vi "Handle Command.vi"(8 "error in":errorcluster, 10 "Change TEC SPs in":refnum<class "Change TEC SPs.lvclass">, 11 "Object In":refnum<class>) -> (0 "error out":errorcluster, 1 "Command Successful?":bool, 2 "Change TEC SPs out":refnum<class "Change TEC SPs.lvclass">, 3 "Object Out":refnum<class>)   [LabVIEW 2014, in "Change TEC SPs.lvclass"]
doc: "Abstract method for accomplishing the execution of a command directed to an instrument object on the wire."
uses:
  Change TEC SPs.lvclass
  Instrument/ePAS.lvclass
  <vilib>/DAQmx/write.llb/DAQmx Write (Analog 1D DBL NChan 1Samp).vi
  reusable/Session APIs/Session Log/System Log.lvclass
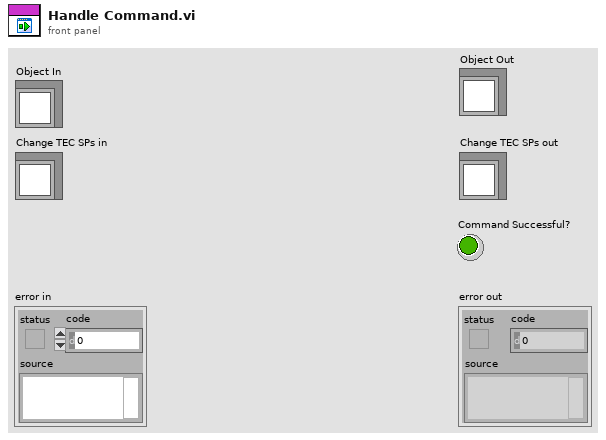
[diagram p1: front panel]
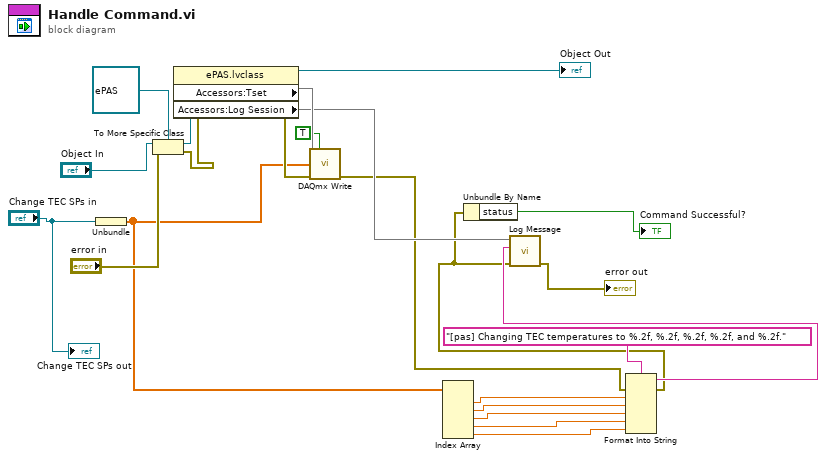
[diagram p0: block diagram]
diagram:
  n1 = Unbundle("Change TEC SPs in") -> (w4:sgl[])
  n2 = To More Specific Class(target class=refnum<class "ePAS.lvclass"> refnum ("ePAS"), reference="Object In", error in="error in") -> (specific class reference=w20:refnum<class "ePAS.lvclass">, error out=w19:errorcluster)
  n3 = property class="ePAS.lvclass"(reference=w20, error in=w19) -> (reference out=→"Object Out":refnum<class "ePAS.lvclass">, error out=w18:errorcluster, "Accessors:Tset"=w17, "Accessors:Log Session"=w16)
  n4 = call-poly <vilib>:"DAQmx Write.vi"("task/channels in"=w17, "auto start"=TRUE, "data"=w4, "error in"=w18) -> ("error out"=w8:errorcluster)  [unwired: 9 in, 2 out]
  n5 = Index Array(array=w4) -> (element #1=w14:sgl, element #2=w13:sgl, element #3=w12:sgl, element #4=w11:sgl, element #5=w10:sgl)  [unwired: 5 in]
  n6 = Format Into String(format string="[pas] Changing TEC temperatures to %.2f, %.2f, %.2f, %.2f, and %.2f.", error in=w8, w14, w13, w12, w11, w10) -> (resulting string=w9:string, error out=w2:errorcluster)  [unwired: 1 in]
  n7 = Unbundle By Name(w2) -> ("status"=→"Command Successful?":bool)
  n8 = call "Log Message.vi"("error in"=w2, "MSG In"=w9, "session in"=w16) -> ("error out"=→"error out":errorcluster)  [unwired: 7 in, 1 out]
  "Change TEC SPs out" <- "Change TEC SPs in"
